vi "MB ICPCON Param Read Ip addr all.vi"(7 "Param Reference":T2, 8 "error in (no error)":errorcluster) -> (0 "error out":errorcluster, 1 "IP address":T1(array[cluster]))   [LabVIEW 2019, in "ICPCON_Param.lvlib"]
uses:
  ICPCON_Param.lvlib
  ICPCON Param.ctl
  Eth timeouts.ctl
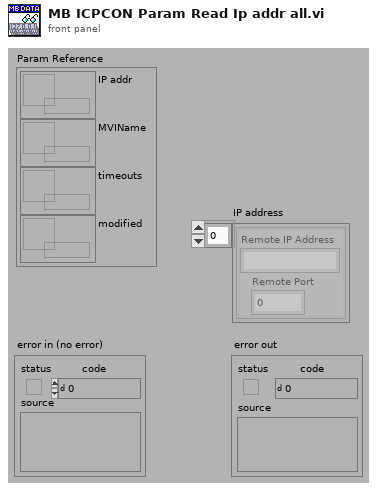
[diagram p1: front panel]
types:
  T1 = cluster{"Remote IP Address":string, "Remote Port":u16}[]
  T2 = typedef "ICPCON_Param.lvlib/ICPCON Param.ctl" = cluster{"IP addr":refnum<data-value>, "MVIName":refnum<data-value>, "timeouts":refnum<data-value>, "modified":refnum<data-value>}
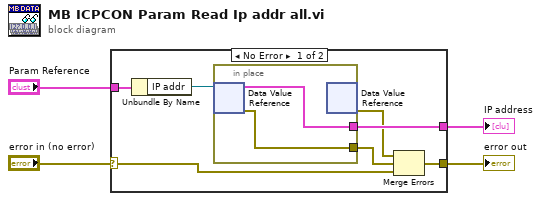
[diagram p0: block diagram]
diagram:
  n1 = case shown="No Error" "error in (no error)" {
    selector: "error in (no error)" -> [w5 w14]
    tunnel: [w9 w14] -> w4
    tunnel: [w11 _] -> w2
    tunnel: "Param Reference" -> [w10 _]
    frame No Error {
      n2 = Unbundle By Name(w10) -> ("IP addr"=w6:refnum<data-value>)
      n3 = in-place {
        in-place-border: [w12] -> w11
        in-place-border: [w13] -> w7
        n4 = in-place-dvr #1(w6) -> (w12:T1, w13:errorcluster)
        n5 = in-place-dvr #1() -> (w8:errorcluster)  [unwired: 1 in, 1 out]
      }
      n6 = Merge Errors(w8, w7, w5) -> (w9:errorcluster)
    }
    frame Error {
    }
  }
  "error out" <- w4
  "IP address" <- w2
